vi "FastArraySumSGL.vi"(4 "2-D data array":sgl[][](array[numeric]), 6 "sample rate MHz":u16, 7 "Type of Mean":T1=enum."No mean", 8 "Bit Depth":i32=8, 9 "Perform Sum?":bool=TRUE, 10 "Filter Prams":T2, 11 "Data Value Reference in":refnum<data-value>) -> (3 "Data Value Reference out":refnum<data-value>)   [LabVIEW 2022 SP3]
uses:
  ViewData/-ReadEye/TypeDefs/TypeofMean.ctl
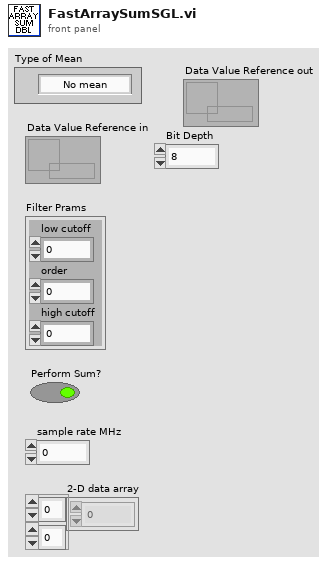
[diagram p1: front panel]
types:
  T1 = typedef "TypeofMean.ctl" = enum16{"Mean from lines", "Mean just lines", "Poly Mean", "No mean", "Filter"}
  T2 = cluster{"low cutoff":i32, "order":i32, "high cutoff":i32}
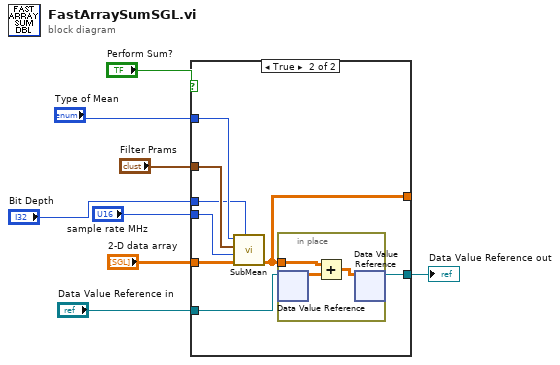
[diagram p0: block diagram]
diagram:
  n1 = case shown="True" "Perform Sum?" {
    tunnel: "Type of Mean" -> [_ w18]
    tunnel: "Filter Prams" -> [_ w17]
    tunnel: "Data Value Reference in" -> [w10 w16]
    tunnel: [w10 w15] -> w5
    tunnel: "2-D data array" -> [w9 w14]
    tunnel: "sample rate MHz" -> [_ w13]
    tunnel: [w9 w12] -> _
    tunnel: "Bit Depth" -> [_ w11]
    frame False {
    }
    frame True {
      n2 = call "SubMean.vi"("Bit Depth"=w11, "Scan Data In"=w14, "Samp Rate (MHz)"=w13, "Filter Prams"=w17, "Type of Mean"=w18) -> ("Array"=w12:dbl[][])  [unwired: 1 in, 2 out]
      n3 = in-place {
        in-place-border: w12 -> [w19]
        n4 = in-place-dvr #1(w16) -> (w21:dbl[][])  [unwired: 1 out]
        n5 = Add(x=w19, y=w21) -> (x+y=w20:dbl[][])
        n6 = in-place-dvr #1(w20) -> (w15:refnum<data-value>)  [unwired: 1 out]
      }
    }
  }
  "Data Value Reference out" <- w5
